vi "Test Log speed.vi"(8 "error in (no error)":errorcluster) -> (0 "error out":errorcluster)   [LabVIEW 2022 SP3]
uses:
  2018adb7-d042-4f93-ad9e-3632fc3fb297.vi
  f4c85acf-a246-4021-baa4-e06f8e43e546.vi
  b532322b-cef8-4434-b98a-5ac6aacd7b76.vi
panel:
  out "second":u32
  out "first":u32
  out "XY Graph":cluster{"timestamps":timestamp[], "data":dbl[]}(graph)
  in  "Current File":path
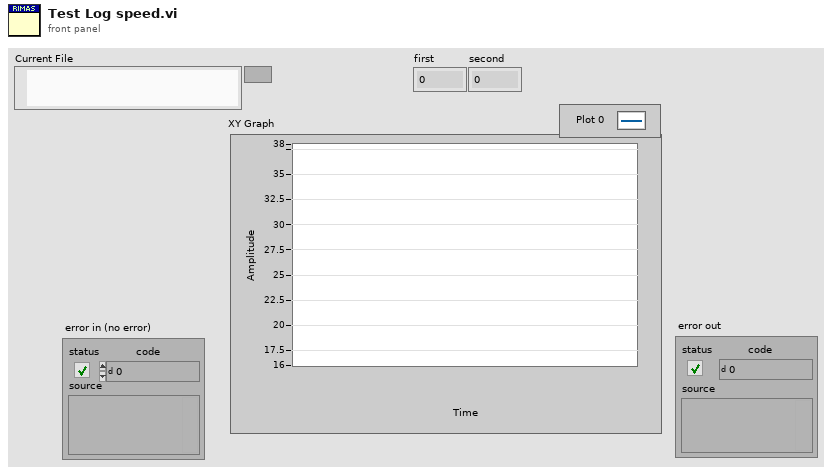
[diagram p1: front panel]
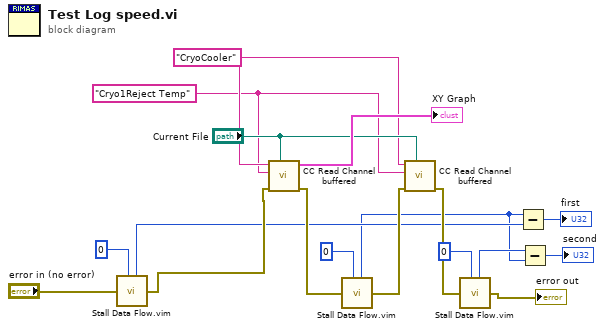
[diagram p0: block diagram]
diagram:
  w4 = "Cryo1Reject Temp" ("group")
  w5 = "CryoCooler" ("group")
  n1 = call "Stall Data Flow.vim"("value in"="error in (no error)", "milliseconds to wait"=u32 0) -> ("millisecond timer value"=w10:u32, "value out"=w17:errorcluster)
  n2 = call "CC Read Channel buffered.vi"("Current File"="Current File", "error in (no error)"=w17, "channel"=w4, "group"=w5) -> ("error out"=w14:errorcluster, "Data"=→"XY Graph":cluster{"timestamps":timestamp[], "data":dbl[]})  [unwired: 5 in, 1 out]
  n3 = call "Stall Data Flow.vim"("value in"=w14, "milliseconds to wait"=u32 0) -> ("millisecond timer value"=w8:u32, "value out"=w13:errorcluster)
  n4 = call "CC Read Channel buffered.vi"("Current File"="Current File", "error in (no error)"=w13, "channel"=w4, "group"=w5) -> ("error out"=w12:errorcluster)  [unwired: 5 in, 2 out]
  n5 = call "Stall Data Flow.vim"("value in"=w12, "milliseconds to wait"=u32 0) -> ("millisecond timer value"=w9:u32, "value out"=→"error out":errorcluster)
  n6 = Subtract(x=w8, y=w10) -> (x-y=→"first":u32)
  n7 = Subtract(x=w9, y=w8) -> (x-y=→"second":u32)
